vi "LVJSON List.vi"(8 "error in (no error)":errorcluster, 11 "Root Element in":T2) -> (0 "error out":errorcluster, 1 "Type":T1, 2 "Keys/Indexes":string[](array[string]), 3 "dup Root Element":T2)   [LabVIEW 2018, in "labview_json.lvlib"]
uses:
  labview_json.lvlib
  Element Type.ctl
  Element.ctl
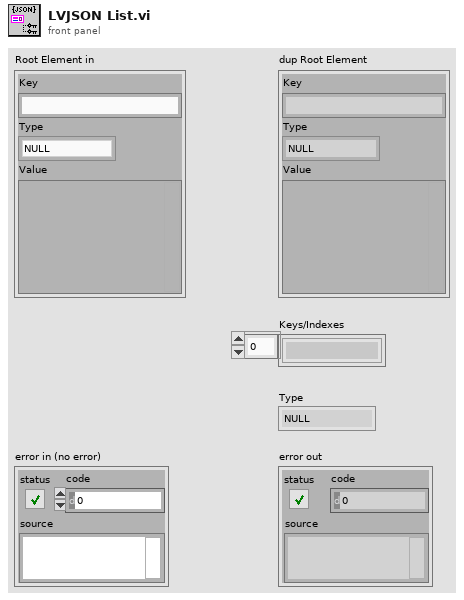
[diagram p1: front panel]
types:
  T1 = typedef "labview_json.lvlib/Element Type.ctl" = enum8{"NULL", "BOOL", "INT", "UINT", "FLOAT", "STRING", "ARRAY", "OBJECT", "SKIP"}
  T2 = typedef "labview_json.lvlib/Element.ctl" = cluster{"Key":string, "Type":T1, "Value":variant}
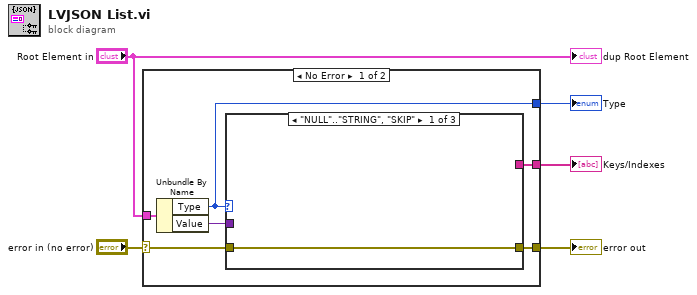
[diagram p0: block diagram]
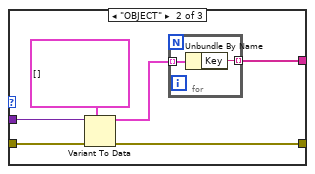
[diagram p2: hidden frame]
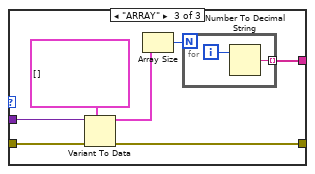
[diagram p3: hidden frame]
diagram:
  n1 = case shown="No Error" "error in (no error)" {
    selector: "error in (no error)" -> [w11 w30]
    tunnel: [w10 w30] -> w4
    tunnel: [w9 _] -> w1
    tunnel: "Root Element in" -> [w8 _]
    tunnel: [w6 _] -> w2
    frame No Error {
      n2 = Unbundle By Name(w8) -> ("Type"=w6:T1, "Value"=w7:variant)
      n3 = case shown="\"NULL\"..\"STRING\", \"SKIP\"" w6 {
        tunnel: w7 -> [_ w18 w27]
        tunnel: w11 -> [w12 w16 w25]
        tunnel: [w12 w15 w24] -> w10
        tunnel: [_ w13 w23] -> w9
        frame "NULL".."STRING", "SKIP" {
        }
        frame "OBJECT" {
          n4 = Variant To Data(error in=w16, type=T2[] [] ("Values"), Variant=w18) -> (data=w14:T2[], error out=w15:errorcluster)
          n5 = for {
            tunnel: w14 -> [w20] mode=indexing
            tunnel: [w19] -> w13 mode=indexing
            n6 = Unbundle By Name(w20) -> ("Key"=w19:string)
          }
        }
        frame "ARRAY" {
          n7 = Variant To Data(error in=w25, type=T2[] [] ("Values"), Variant=w27) -> (data=w22:T2[], error out=w24:errorcluster)
          n8 = Array Size(array=w22) -> (size(s)=w21:i32)
          n9 = for {
            N: w21 -> [_]
            tunnel: [w28] -> w23 mode=indexing
            i -> [w29]
            n10 = Number To Decimal String(number=w29) -> (decimal integer string=w28:string)  [unwired: 1 in]
          }
        }
      }
    }
    frame Error {
    }
  }
  "error out" <- w4
  "Keys/Indexes" <- w1
  "Type" <- w2
  "dup Root Element" <- "Root Element in"
